vi "Init_.vi"(8 "error in (no error)":errorcluster, 9 "lib":string="RT_Shared_Variables", 10 "host":string="localhost") -> (0 "error out":errorcluster, 3 "SV_Publisher out":refnum<class "SV_Publisher.lvclass">)   [LabVIEW 2019, in "SV_Publisher.lvclass"]
uses:
  SV_Publisher.lvclass
  Data.ctl
  SV_Publisher.lvclass/SV_Publisher.ctl
  SV_Wrap/SharedVariableWrapper.lvclass
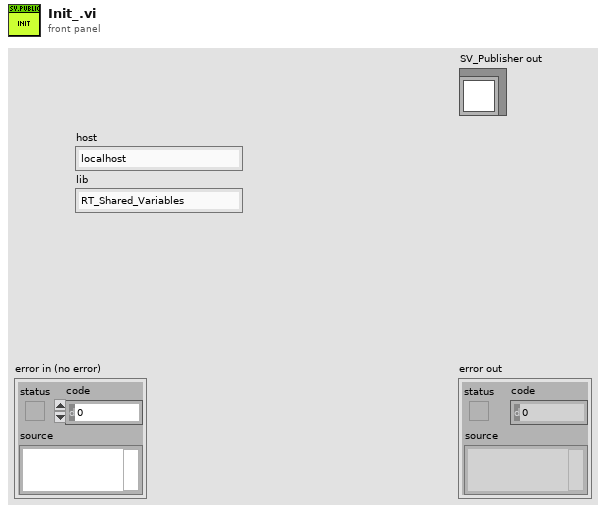
[diagram p1: front panel]
types:
  T1 = typedef "SV_Publisher.lvclass/Data.ctl" = cluster{"Name":string, "Value":variant}
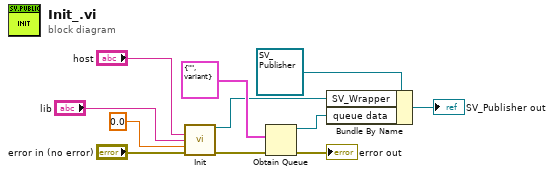
[diagram p0: block diagram]
diagram:
  n1 = call "Init.vi"("host"="host", "lib"="lib", "update timeout"=0.0, "error in (no error)"="error in (no error)") -> ("SVW"=w4:refnum<class "SharedVariableWrapper.lvclass">, "error out"=w3:errorcluster)  [unwired: 10 in]
  n2 = Obtain Queue(element data type=T1 {"Name"="", "Value"=variant} ("Data"), error in (no error)=w3) -> (queue out=w1:refnum<queue>, error out=→"error out":errorcluster)  [unwired: 3 in, 1 out]
  n3 = Bundle By Name(cluster=refnum<class "SV_Publisher.lvclass"> refnum ("SV_Publisher in"), "SV_Wrapper"=w4, "queue data"=w1) -> (→"SV_Publisher out":refnum<class "SV_Publisher.lvclass">)
